vi "Read XML_Extra Checks_Check Parameter Name Uniqueness.vi"(8 "error in (no error)":errorcluster, 11 "Channels In":T1[](array[typedef])) -> (0 "error out":errorcluster)   [LabVIEW 2019]
doc: "This VI checks that for a given Hardware Channel, all parameters have a unique combination of Parameter settings: Hardware Channel, Label Decimal and Parameter Name. If there are multiple duplicates, the function returns all duplicates."
uses:
  XML_Channel.ctl
  XML_Label.ctl
  XML_Parameter.ctl
  <userlib>/_OpenG.lib/md5/md5.llb/MD5 Message Digest (Binary String)__ogtk.vi
  <userlib>/_OpenG.lib/array/array.llb/Remove Duplicates from 1D Array (String)__ogtk.vi
panel:
  out "Error Source":string
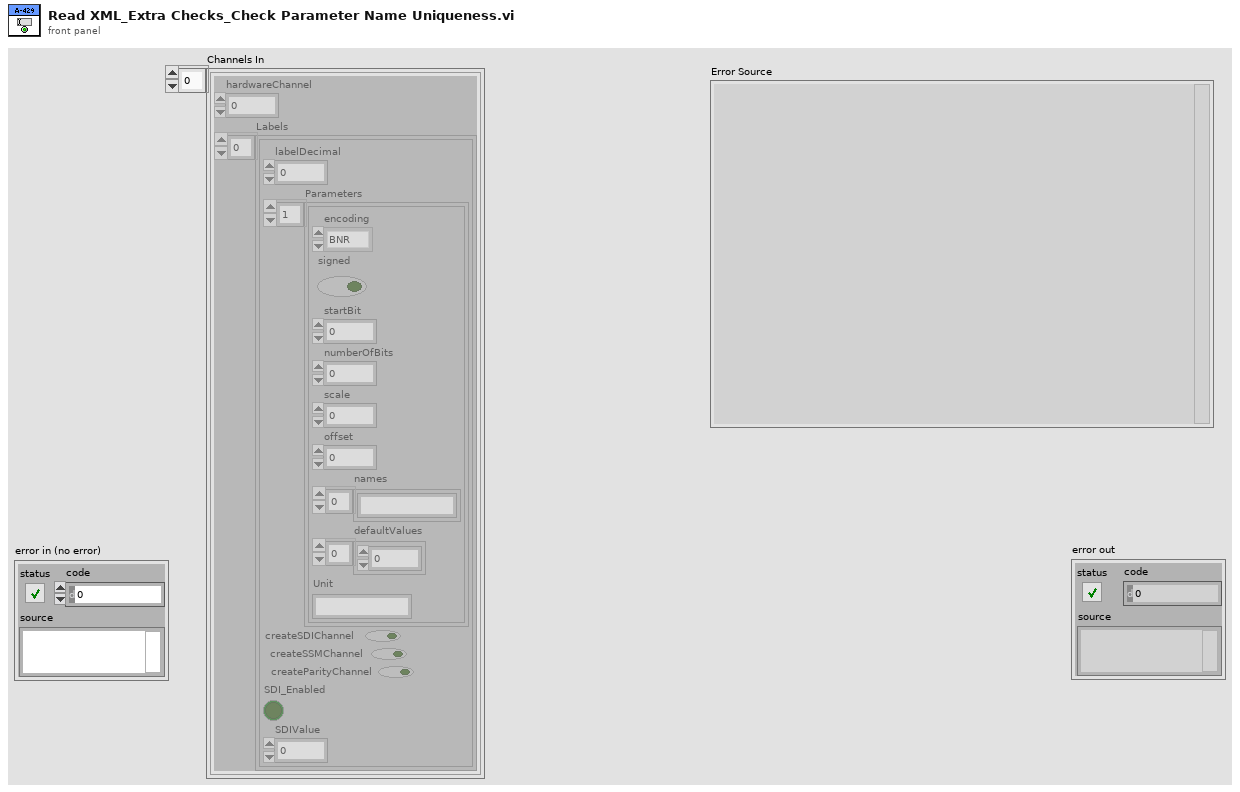
[diagram p1: front panel]
types:
  T1 = typedef "XML_Channel.ctl" = cluster{"hardwareChannel":i32, "Labels":T2[]}
  T2 = typedef "XML_Label.ctl" = cluster{"labelDecimal":i32, "Parameters":T3[], "createSDIChannel":bool, "createSSMChannel":bool, "createParityChannel":bool, "SDI_Enabled":bool, "SDIValue":u8}
  T3 = typedef "XML_Parameter.ctl" = cluster{"encoding":enum16{"BNR", "BCD", "Discrete"}, "signed":bool, "startBit":i32, "numberOfBits":i32, "scale":dbl, "offset":dbl, "names":string[], "defaultValues":dbl[], "Unit":string}
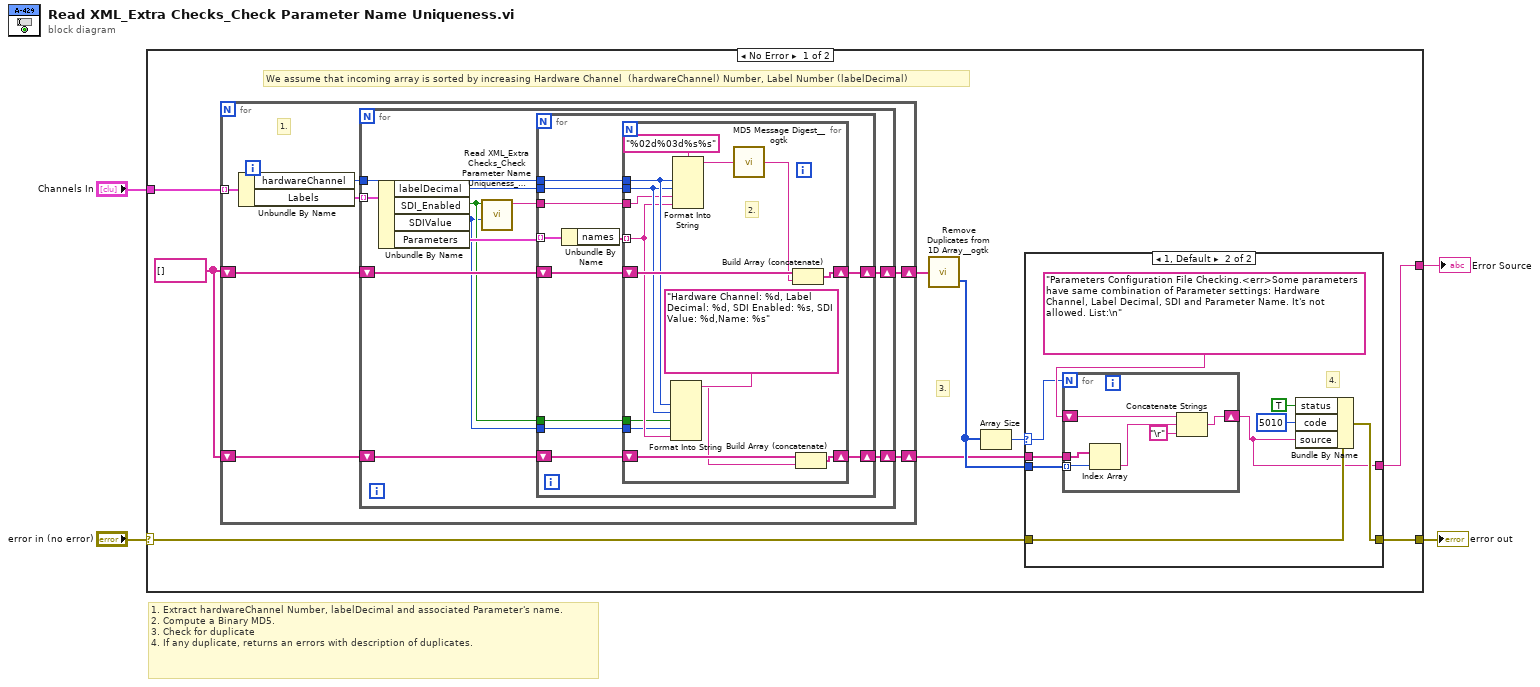
[diagram p0: block diagram]
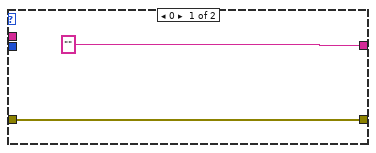
[diagram p2: hidden frame]
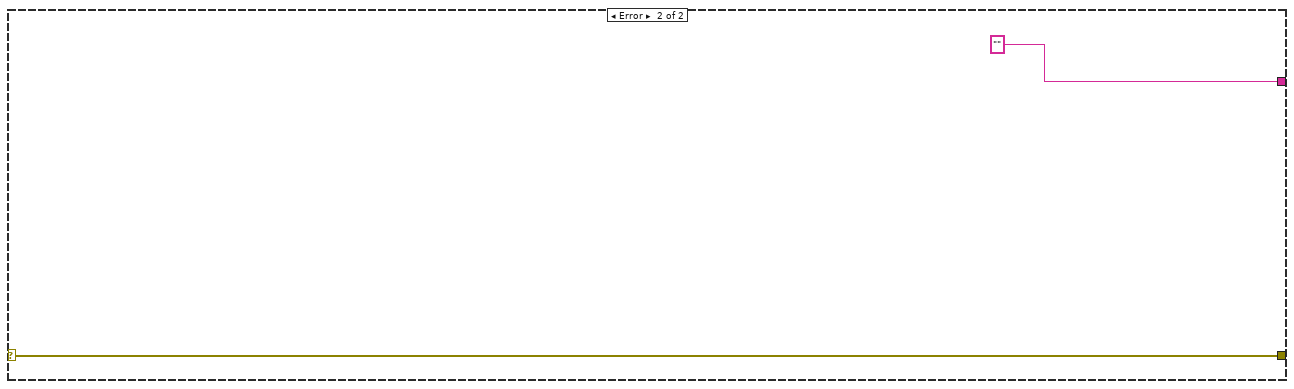
[diagram p3: hidden frame]
diagram:
  # "1. Extract hardwareChannel Number, labelDecimal and associated Parameter's name.\n2. Compute a Binary MD5.\n3. Check for duplicate\n4. If any duplicate, returns an errors with description of duplicates."
  n1 = case shown="No Error" "error in (no error)" {
    selector: "error in (no error)" -> [w12 w76]
    tunnel: [w9 w76] -> w3
    tunnel: "Channels In" -> [w11 _]
    tunnel: [w8 ""] -> w1
    frame No Error {
      w6 = string[] []
      # "3."
      # "We assume that incoming array is sorted by increasing Hardware Channel  (hardwareChannel) Number, Label Number (labelDecimal)"
      n2 = for {
        tunnel: w11 -> [w37] mode=indexing
        shift-right: [w33] -> w7
        shift-left: w6 -> [w34]
        shift-right: [w31] -> w5
        shift-left: w6 -> [w32]
        # "1."
        n3 = Unbundle By Name(w37) -> ("hardwareChannel"=w36:i32, "Labels"=w35:T2[])
        n4 = for {
          tunnel: w36 -> [w48]
          tunnel: w35 -> [w47] mode=indexing
          shift-right: [w44] -> w33
          shift-left: w34 -> [w45]
          shift-right: [w42] -> w31
          shift-left: w32 -> [w43]
          n5 = Unbundle By Name(w47) -> ("labelDecimal"=w46:i32, "SDI_Enabled"=w39:bool, "SDIValue"=w38:u8, "Parameters"=w41:T3[])
          n6 = call "Read XML_Extra Checks_Check Parameter Name Uniqueness_create SDI string.vi"("SDIValue"=w38, "SDI_Enabled"=w39) -> ("SDI String"=w40:string)  [unwired: 9 in]
          n7 = for {
            tunnel: w48 -> [w59]
            tunnel: w46 -> [w58]
            shift-right: [w56] -> w44
            shift-left: w45 -> [w57]
            tunnel: w41 -> [w55] mode=indexing
            shift-right: [w52] -> w42
            shift-left: w43 -> [w53]
            tunnel: w40 -> [w51]
            tunnel: w39 -> [w50]
            tunnel: w38 -> [w49]
            n8 = Unbundle By Name(w55) -> ("names"=w54:string[])
            n9 = for {
              tunnel: w59 -> [w67]
              tunnel: w58 -> [w66]
              tunnel: w54 -> [w62] mode=indexing
              shift-right: [w71] -> w56
              shift-left: w57 -> [w72]
              shift-right: [w68] -> w52
              shift-left: w53 -> [w69]
              tunnel: w51 -> [w63]
              tunnel: w50 -> [w61]
              tunnel: w49 -> [w60]
              # "2."
              n10 = Format Into String(format string="Hardware Channel: %d, Label Decimal: %d, SDI Enabled: %s, SDI Value: %d,Name: %s", w67, w66, w61, w60, w62) -> (resulting string=w64:string)  [unwired: 2 in, 1 out]
              n11 = Format Into String(format string="%02d%03d%s%s", w67, w66, w63, w62) -> (resulting string=w73:string)  [unwired: 2 in, 1 out]
              n12 = call-poly <userlib>:"MD5 Message Digest__ogtk.vi"("Message"=w73) -> ("MD5 Message Digest"=w70:string)
              n13 = Build Array (concatenate)(w72, w70) -> (w71:string[])
              n14 = Build Array (concatenate)(w69, w64) -> (w68:string[])
            }
          }
        }
      }
      n15 = call-poly <userlib>:"Remove Duplicates from 1D Array__ogtk.vi"("Input Array"=w7) -> ("indices of removed elements"=w10:i32[])  [unwired: 1 out]
      n16 = Array Size(array=w10) -> (size(s)=w13:i32)
      n17 = case shown="1, Default" w13 {
        selector: w13 -> [_ w19]
        tunnel: w12 -> [w15 w24]
        tunnel: w10 -> [_ w18]
        tunnel: [w15 w23] -> w9
        tunnel: ["" w17] -> w8
        tunnel: w5 -> [_ w16]
        frame 0 {
        }
        frame 1, Default {
          # "4."
          n18 = for {
            N: w19 -> [_]
            shift-right: [w29] -> w17
            shift-left: "Parameters Configuration File Checking.<err>Some parameters have same combination of Parameter settings: Hardware Channel, Label Decimal, SDI and Parameter Name. It's not allowed. List:\n" -> [w30]
            tunnel: w18 -> [w28] mode=indexing
            tunnel: w16 -> [w26]
            n19 = Index Array(array=w26, index=w28) -> (element=w25:string)
            n20 = Concatenate Strings(w30, w25, "\r") -> (w29:string)
          }
          n21 = Bundle By Name(cluster=w24, "status"=TRUE, "code"=5010, "source"=w17) -> (w23:errorcluster)
        }
      }
    }
    frame Error {
    }
  }
  "error out" <- w3
  "Error Source" <- w1
